vi "PPS TCP Parser's Calling or Specified VI's Clustered Controls Details.vi"(0 "Calling VI (T)":bool, 5 "Specified VI (if Calling VI = F)":path=path "Optical Prober Control v5.0.2j.vi", 11 "error in (no error)":errorcluster) -> (1 "Direct-access\ncontrols for\nrelabeling":refnum<vi>[](array[refnum]), 2 "Refs to controls on panel":refnum<vi>[](array[refnum]), 3 "Direct-access\ncontrols for\nrelabeling: captions":string[](array[string])=["Application Directory", "Direct Name 1", "Direct Position 1", "Direct Jog - 1", "Direct Jog + 1", "Direct Step (mm) 1", "Direct Halt Axis 1", "Direct Settings 1", "Direct Moving 1", "Direct New target 1", "Direct OK 1", "Direct Home Axis 1", "Direct Home Axis 2", "Direct OK 2", "Direct New target 2", "Direct Moving 2", "Direct Settings 2", "Direct Halt Axis 2", "Direct Step (mm) 2", "Direct Jog + 2", "Direct Jog - 2", "Direct Position 2", "Direct Name 2", "Direct Home Axis 3", "Direct OK 3", "Direct New target 3", "Direct Moving 3", "Direct Settings 3", "Direct Halt Axis 3", "Direct Step (mm) 3", "Direct Jog + 3", "Direct Jog - 3", "Direct Position 3", "Direct Name 3", "Direct Home Axis 4", "Direct OK 4", "Direct New target 4", "Direct Moving 4", "Direct Settings 4", "Direct Halt Axis 4", "Direct Step (mm) 4", "Direct Jog + 4", "Direct Jog - 4", "Direct Position 4", "Direct Name 4", "Direct Home Axis 5", "Direct OK 5", "Direct New target 5", "Direct Moving 5", "Direct Settings 5", "Direct Halt Axis 5", "Direct Step (mm) 5", "Direct Jog + 5", "Direct Jog - 5", "Direct Position 5", "Direct Name 5", "Direct Home Axis 6", "Direct OK 6", "Direct New target 6", "Direct Moving 6", "Direct Settings 6", "Direct Halt Axis 6", "Direct Step (mm) 6", "Direct Jog + 6", "Direct Jog - 6", "Direct Position 6", "Direct Name 6"], 4 "Names of Clusters":string[](array[string])=["error out"], 6 "Controls in\nthose clusters":string[][](array[string])=[["status", "code", "source"]], 8 "Refs to controls in clusters":refnum<vi>[][](array[refnum]), 10 "Refs to clusters":refnum<vi>[](array[refnum]), 12 "Controls directly on tab panes":string[](array[string])=["Interface", "S/N", "System no.", "Input XY bulls-eye", "Output XY bulls-eye", "Input Z bulls-eye", "RS Start", "RS Input XY:Enable", "RS Output XY:Enable", "RS Input XY:Status", "RS Output XY:Status", "RS Display Raw Data", "RS Input X:Range", "RS Input Y:Range", "RS Input Y:Step", "GS Start", "GS Display Raw Data", "I(t)", "Power Meter", "Output Z bulls-eye", "stop", "ID", "RS Frequency", "RS Input X:Center", "RS Input Y:Center", "RS Output X:Range", "RS Output Y:Range", "RS Output Y:Step", "RS Output X:Center", "RS Output Y:Center", "RS Input XY:Duration", "RS Output XY:Duration", "idle loop (msec)", "RS:Settle at 1st corner", "Axis role file", "Application Directory", "GS Status", "Power Meter Average", "RS Input XY:Swap Axes", "RS Output XY:Swap Axes", "PZT Input X:Position", "PZT Input Y:Position", "PZT Output X:Position", "PZT Output Y:Position", "PZT Input Z:Position", "PZT Output Z:Position", "RS Status", "PZT motion", "Motor motion", "Motor Input X:Name", "Motor Input X:Position", "Motor Input X:Jog +", "Motor Input X:Jog -", "Motor Input X:Step (mm)", "Motor Input X:Halt Axis", "Motor Input X:Settings", "Motor Input X:Moving", "Motor Input X:New Target", "Motor Input X:OK", "Motor Input X:Home Axis", "Motor Input Y:Home Axis", "Motor Input Y:OK", "Motor Input Y:New Target", "Motor Input Y:Moving", "Motor Input Y:Settings", "Motor Input Y:Halt Axis", "Motor Input Y:Step (mm)", "Motor Input Y:Jog -", "Motor Input Y:Jog +", "Motor Input Y:Position", "Motor Input Y:Name", "Motor Input Z:Home Axis", "Motor Input Z:OK", "Motor Input Z:New Target", "Motor Input Z:Moving", "Motor Input Z:Settings", "Motor Input Z:Halt Axis", "Motor Input Z:Step (mm)", "Motor Input Z:Jog -", "Motor Input Z:Jog +", "Motor Input Z:Position", "Motor Input Z:Name", "Motor Output X:Home Axis", "Motor Output X:OK", "Motor Output X:New Target", "Motor Output X:Moving", "Motor Output X:Settings", "Motor Output X:Halt Axis", "Motor Output X:Step (mm)", "Motor Output X:Jog -", "Motor Output X:Jog +", "Motor Output X:Position", "Motor Output X:Name", "Motor Output Y:Home Axis", "Motor Output Y:OK", "Motor Output Y:New Target", "Motor Output Y:Moving", "Motor Output Y:Settings", "Motor Output Y:Halt Axis", "Motor Output Y:Step (mm)", "Motor Output Y:Jog -", "Motor Output Y:Jog +", "Motor Output Y:Position", "Motor Output Y:Name", "Motor Output Z:Home Axis", "Motor Output Z:OK", "Motor Output Z:New Target", "Motor Output Z:Moving", "Motor Output Z:Settings", "Motor Output Z:Halt Axis", "Motor Output Z:Step (mm)", "Motor Output Z:Jog -", "Motor Output Z:Jog +", "Motor Output Z:Position", "Motor Output Z:Name", "GS Input XY:Enable", "GS Output XY:Enable", "GS Input Z:Enable", "GS Output Z:Enable", "GS Input XY:Status", "GS Output XY:Status", "GS Input Z:Status", "GS Output Z:Status", "RS Fit", "RS:Lower Clip Level", "RS:Upper Clip Level", "GS:Couple Processes", "FW", "RS Input:Successful", "GS Input XY:Success", "GS Output XY:Success", "GS Input Z:Success", "GS Output Z:Success", "RS Input:Threshold (mW)", "RS Output:Threshold (mW)", "RS Output:Successful", "Default settling window", "Scan axis center", "Step axis center", "Z axis center", "NxM Dithers", "RS Input XY:Data", "RS Output XY:Data", "error out", "Override Pane", "GS Input XY:Duration", "GS Output XY:Duration", "GS Input Z:Duration", "GS Input Z:Duration", "PZT Input X:New Target", "Scan Processes (from axis roles file)", "GS Parameters:Update", "PZT Input Y:New Target", "PZT Output X:New Target", "PZT Output Y:New Target", "PZT Output Z:New Target", "PZT Input Z:New Target", "GS Input XY:HZ", "GS Input XY:V", "GS Input XY:MDC", "GS Input XY:MINR", "GS Input XY:MAXR", "GS Input XY:ML", "GS Input XY:SP", "GS Output XY:HZ", "GS Output XY:V", "GS Output XY:MDC", "GS Output XY:MINR", "GS Output XY:MAXR", "GS Output XY:ML", "GS Output XY:SP", "GS Input Z:HZ", "GS Input Z:V", "GS Input Z:MDC", "GS Input Z:MINR", "GS Input Z:MAXR", "GS Input Z:ML", "GS Input Z:SP", "GS Output Z:HZ", "GS Output Z:V", "GS Output Z:MDC", "GS Output Z:MINR", "GS Output Z:MAXR", "GS Output Z:ML", "GS Output Z:SP", "GS Input XY process name", "GS Input XY StepAxNumber", "GS Input XY ScanAxNumber", "GS Input XY ScanAxName", "GS Input XY StepAxName", "GS Output XY process name", "GS Output XY StepAxNumber", "GS Output XY ScanAxNumber", "GS Output XY ScanAxName", "GS Output XY StepAxName", "GS Input Z process name", "GS Input Z StepAxNumber", "GS Input Z ScanAxNumber", "GS Input Z ScanAxName", "GS Input Z StepAxName", "GS Output Z process name", "GS Output Z StepAxNumber", "GS Output Z ScanAxNumber", "GS Output Z ScanAxName", "GS Output Z StepAxName", "msec timestamp"], 13 "Refs to controls directly on tab panes":refnum<vi>[](array[refnum]), 14 "Controls on panel":string[](array[string])=["Halt Homing", "Tab Control", "Names of Clusters", "Controls in clusters", "Refs to clusters", "PZT Input X:OK", "PZT Input Y:OK", "PZT Input Z:OK", "PZT Output X:OK", "PZT Output Y:OK", "PZT Output Z:OK"], 15 "error out":errorcluster)   [LabVIEW 2016]
panel:
  out "Array":string[](array[string])=["Array", "Array", "Array"]
  out "Arrays":string[](array[string])=["Names of Clusters", "Controls in clusters", "Refs to clusters"]
  out "Refs to arrays":refnum<vi>[](array[refnum])
  out "Names of TabControls":string[](array[string])=["Tab Control"]
  out "Refs to TabControls":refnum<vi>[](array[refnum])
  out "Types of Controls\non panel":string[](array[string])=["Boolean", "TabControl", "Array", "Array", "Array", "Boolean", "Boolean", "Boolean", "Boolean", "Boolean", "Boolean"]
  # "This subVI finds the controls that exist on the front panel of the calling VI (OR a \nspecified VI), then selects just-the-clusters from that list.  It then finds the elements of each cluster.\n\nIF the calling VI has tab controls, the structure of this VI must accommodate the number of pages for each tab control.  Here we have nine configurations: 2-10 pages.  Add to these as necessary to accommodate the configuration of the calling VI.\n\nThis VI does not handle calling VIs with tab controls containing tab controls containing clusters...\n\nSee further discussion in the block diagram."
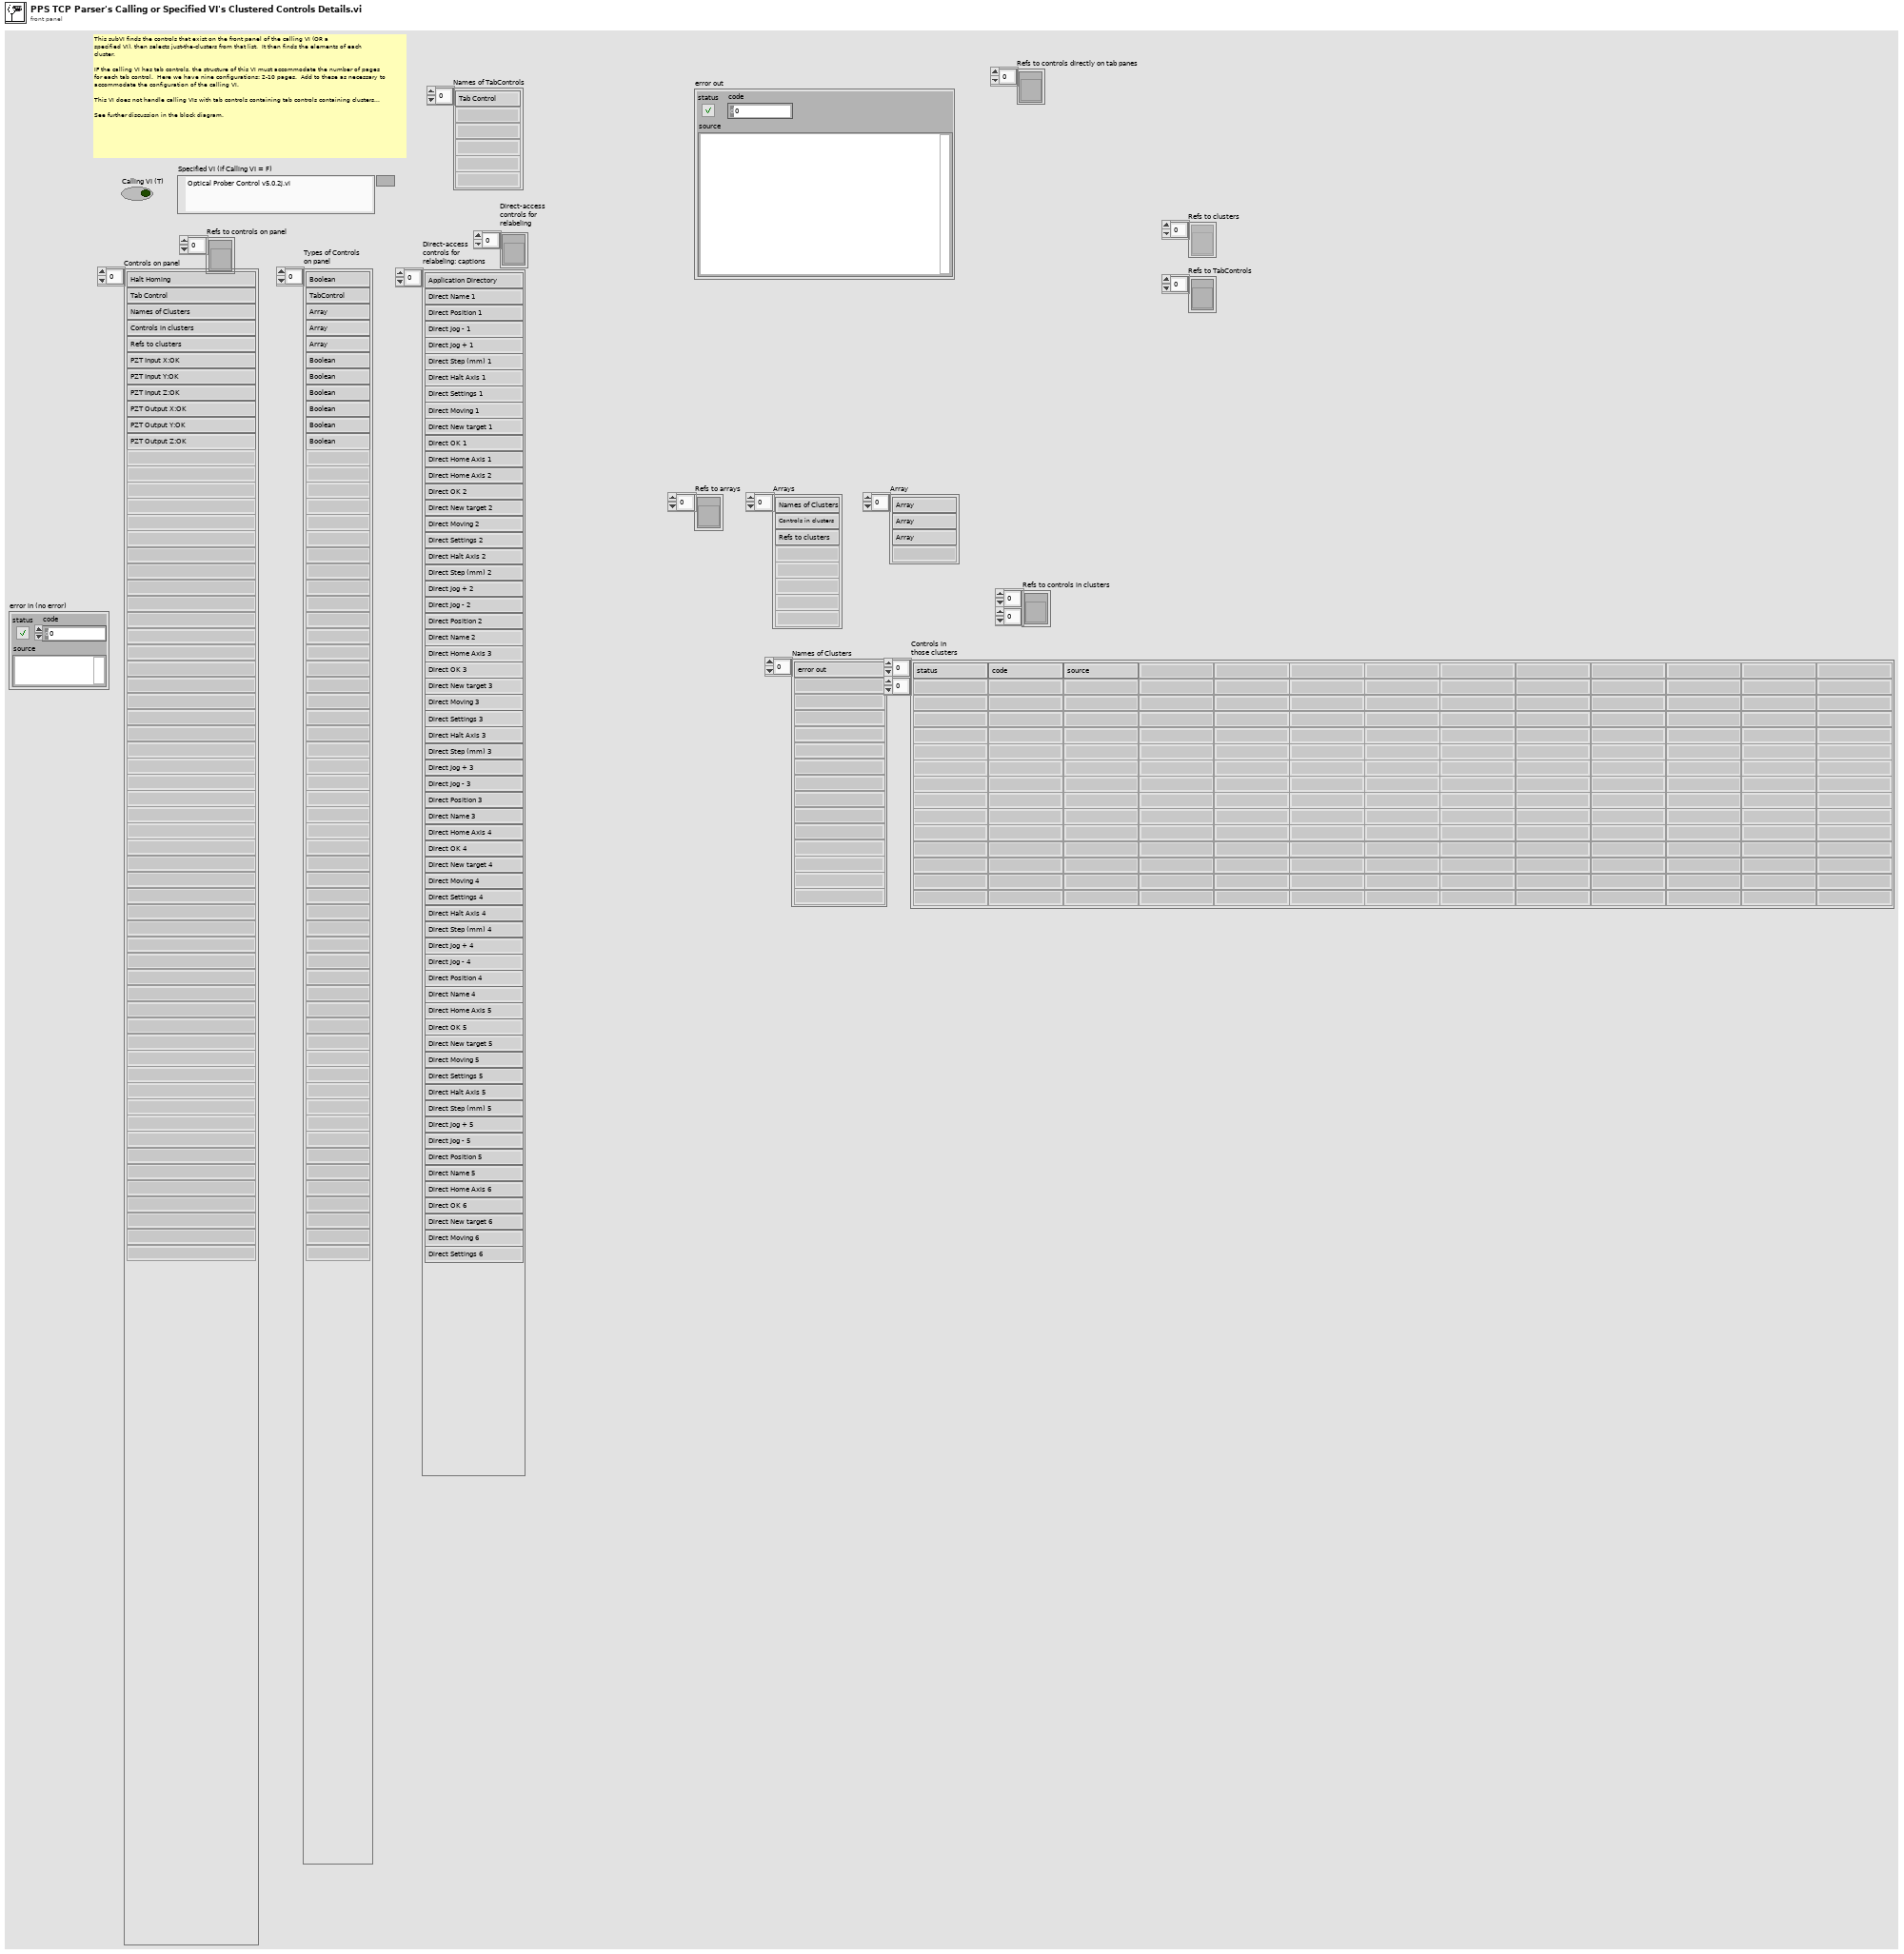
[diagram p1: front panel]
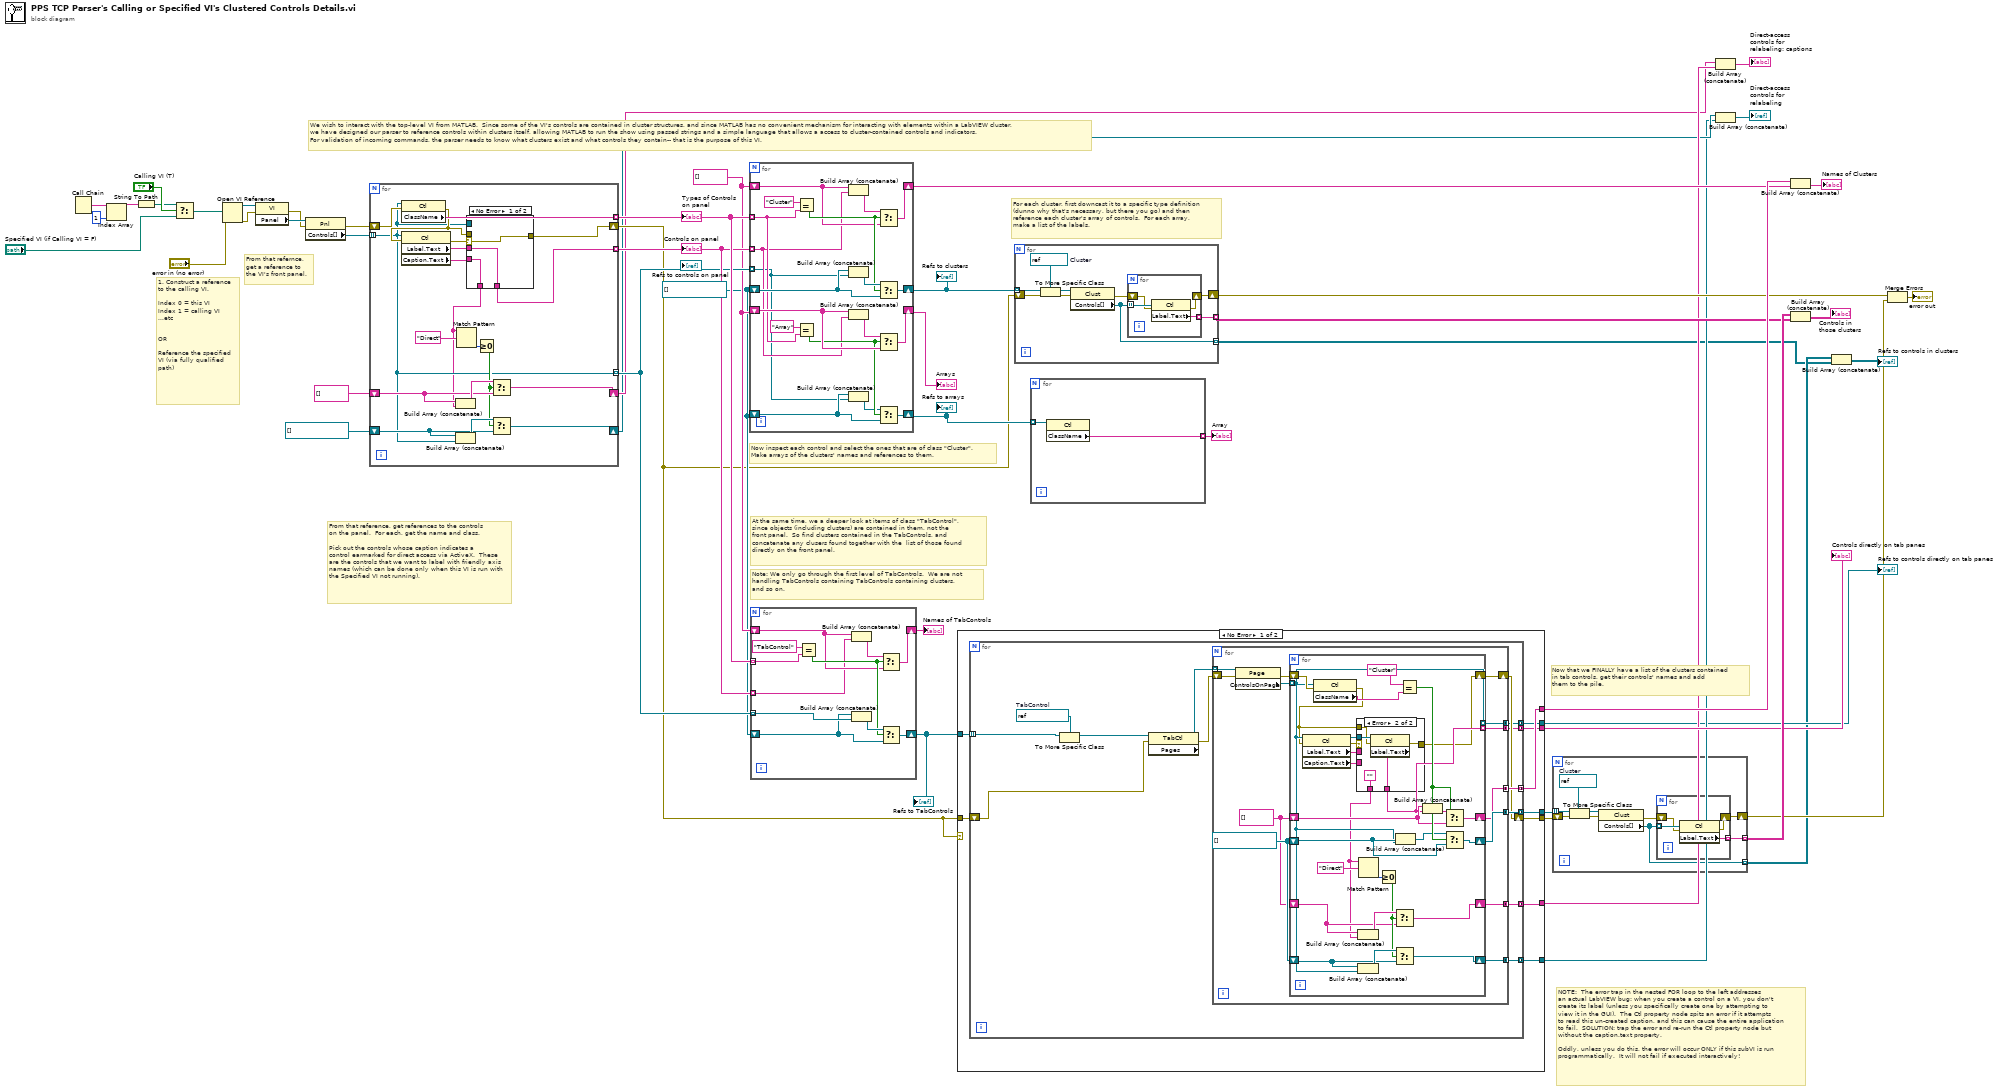
[diagram p0: block diagram]
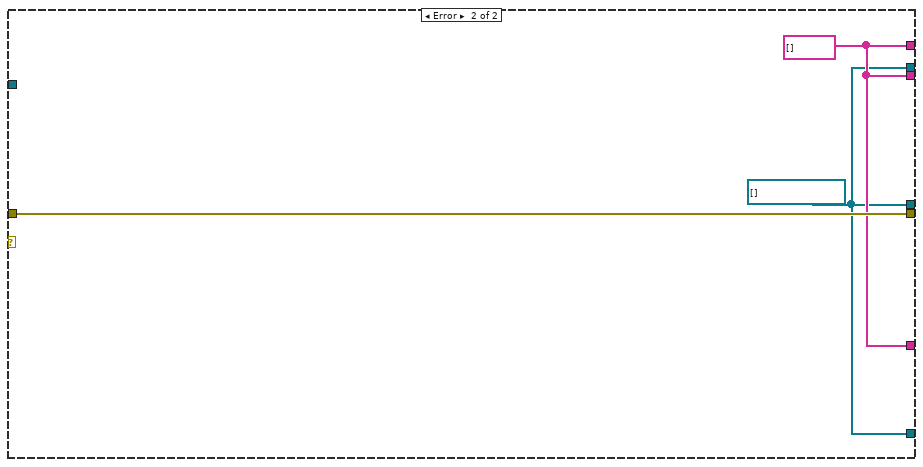
[diagram p3: hidden frame]
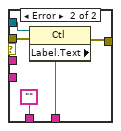
[diagram p4: hidden frame]
diagram:
  w23 = refnum<vi>[] []
  w24 = string[] []
  # "NOTE:  The error trap in the nested FOR loop to the left addresses\nan actual LabVIEW bug: when you create a control on a VI, you don't\ncreate its label (unless you specifically create one by attempting to \nview it in the GUI).  The Ctl property node spits an error if it attempts \nto read this un-created caption, and this can cause the entire application\nto fail.  SOLUTION: trap the error and re-run the Ctl property node but\nwithout the caption.text property.\n\nOddly, unless you do this, the error will occur ONLY if this subVI is run\nprogrammatically.  It will not fail if executed interactively!"
  # "We wish to interact with the top-level VI from MATLAB.  Since some of the VI's controls are contained in cluster structures, and since MATLAB has no convenient mechanism for interacting with elements within a LabVIEW cluster, \nwe have designed our parser to reference controls within clusters itself, allowing MATLAB to run the show using passed strings and a simple language that allows a access to cluster-contained controls and indicators.  \nFor validation of incoming commands, the parser needs to know what clusters exist and what controls they contain-- that is the purpose of this VI."
  # "Now that we FINALLY have a list of the clusters contained\nin tab controls, get their controls' names and add \nthem to the pile."
  # "Note: We only go through the first level of TabControls.  We are not\nhandling TabControls containing TabControls containing clusters,\nand so on."
  # "At the same time, we a deeper look at items of class \"TabControl\", \nsince objects (including clusters) are contained in them, not the\nfront panel.  So find clusters contained in the TabControls, and \nconcatenate any clusers found together with the  list of those found \ndirectly on the front panel."
  # "For each cluster, first downcast it to a specific type definition\n(dunno why that's necessary, but there you go) and then\nreference each cluster's array of controls.  For each array,\nmake a list of the labels."
  # "Now inspect each control and select the ones that are of class \"Cluster\".\nMake arrays of the clusters' names and references to them."
  # "From that reference, get references to the controls\non the panel.  For each, get the name and class.\n\nPick out the controls whose caption indicates a \ncontrol earmarked for direct access via ActiveX.  These are the controls that we want to label with friendly axis names (which can be done only when this VI is run with the Specified VI not running)."
  # "From that refernce,\nget a reference to\nthe VI's front panel."
  # "1. Construct a reference\nto the calling VI.  \n\nIndex 0 = this VI\nIndex 1 = calling VI\n...etc\n\n\nOR\n\nReference the specified\nVI (via fully qualified\npath)"
  n1 = Call Chain() -> (call chain=w47:string[])
  n2 = Index Array(array=w47, index=1) -> (element=w18:string)
  n3 = String To Path(string=w18) -> (path=w15:path)
  n4 = Select(t=w15, s="Calling VI (T)", f="Specified VI (if Calling VI = F)") -> (s? t:f=w17:path)
  n5 = Open VI Reference(vi path=w17, error in (no error)="error in (no error)") -> (vi reference=w45:refnum<vi>, error out=w43:errorcluster)  [unwired: 4 in]
  n6 = property class="VI"(reference=w45, error in=w43) -> (error out=w42:errorcluster, "Panel"=w50:refnum<vi>)  [unwired: 1 out]
  n7 = property class="Pnl"(reference=w50, error in=w42) -> (error out=w41:errorcluster, "Controls[]"=w49:refnum<vi>[])  [unwired: 1 out]
  n8 = for {
    tunnel: w49 -> [w55] mode=indexing
    tunnel: [w52] -> w38 mode=indexing
    tunnel: [w69] -> w39 mode=indexing
    tunnel: [w55] -> w37 mode=indexing
    shift-right: [w57] -> w11
    shift-left: w41 -> [w68]
    shift-right: [w67] -> w9
    shift-left: string[] [] -> [w65]
    shift-right: [w63] -> w7
    shift-left: refnum<vi>[] [] -> [w62]
    n9 = property class="Ctl"(reference=w55, error in=w68) -> (error out=w56:errorcluster, "ClassName"=w69:string)  [unwired: 1 out]
    n10 = property class="Ctl"(reference=w55, error in=w56) -> (error out=w58:errorcluster, "Label.Text"=w54:string, "Caption.Text"=w53:string)  [unwired: 1 out]
    n11 = Build Array (concatenate)(w62, w55) -> (w64:refnum<vi>[])
    n12 = case shown="No Error" w58 {
      selector: w58 -> [w71 _]
      tunnel: w56 -> [_ w73]
      tunnel: w54 -> [w72 _]
      tunnel: [w72 w77] -> w52
      tunnel: w55 -> [_ w74]
      tunnel: [w71 w75] -> w57
      tunnel: [w70 ""] -> w51
      tunnel: w53 -> [w70 _]
      frame No Error {
      }
      frame Error {
        n13 = property class="Ctl"(reference=w74, error in=w73) -> (error out=w75:errorcluster, "Label.Text"=w77:string)  [unwired: 1 out]
      }
    }
    n14 = Build Array (concatenate)(w65, w51) -> (w66:string[])
    n15 = Match Pattern(string=w51, regular expression="Direct") -> (offset past match=w60:i32)  [unwired: 1 in, 3 out]
    n16 = Greater Or Equal To 0?(x=w60) -> (x >= 0?=w59:bool)
    n17 = Select(t=w66, s=w59, f=w65) -> (s? t:f=w67:string[])
    n18 = Select(t=w64, s=w59, f=w62) -> (s? t:f=w63:refnum<vi>[])
  }
  "Controls on panel" <- w38
  "Types of Controls\non panel" <- w39
  "Refs to controls on panel" <- w37
  n19 = for {
    tunnel: w39 -> [w81] mode=indexing
    tunnel: w38 -> [w80] mode=indexing
    shift-right: [w94] -> w31
    shift-left: w24 -> [w90]
    tunnel: w37 -> [w79] mode=indexing
    shift-right: [w92] -> w48
    shift-left: w23 -> [w89]
    shift-right: [w78] -> w22
    shift-left: w24 -> [w87]
    shift-right: [w85] -> w21
    shift-left: w23 -> [w88]
    n20 = Equal?(x="Cluster", y=w81) -> (x = y?=w91:bool)
    n21 = Equal?(x="Array", y=w81) -> (x = y?=w86:bool)
    n22 = Build Array (concatenate)(w90, w80) -> (w95:string[])
    n23 = Build Array (concatenate)(w89, w79) -> (w93:refnum<vi>[])
    n24 = Build Array (concatenate)(w87, w80) -> (w83:string[])
    n25 = Build Array (concatenate)(w88, w79) -> (w84:refnum<vi>[])
    n26 = Select(t=w95, s=w91, f=w90) -> (s? t:f=w94:string[])
    n27 = Select(t=w93, s=w91, f=w89) -> (s? t:f=w92:refnum<vi>[])
    n28 = Select(t=w83, s=w86, f=w87) -> (s? t:f=w78:string[])
    n29 = Select(t=w84, s=w86, f=w88) -> (s? t:f=w85:refnum<vi>[])
  }
  "Refs to clusters" <- w48
  "Refs to arrays" <- w21
  "Arrays" <- w22
  n30 = for {
    tunnel: w39 -> [w107] mode=indexing
    tunnel: w38 -> [w99] mode=indexing
    shift-right: [w104] -> w40
    shift-left: w24 -> [w100]
    tunnel: w37 -> [w98] mode=indexing
    shift-right: [w102] -> w36
    shift-left: w23 -> [w97]
    n31 = Equal?(x="TabControl", y=w107) -> (x = y?=w101:bool)
    n32 = Build Array (concatenate)(w100, w99) -> (w105:string[])
    n33 = Build Array (concatenate)(w97, w98) -> (w103:refnum<vi>[])
    n34 = Select(t=w105, s=w101, f=w100) -> (s? t:f=w104:string[])
    n35 = Select(t=w103, s=w101, f=w97) -> (s? t:f=w102:refnum<vi>[])
  }
  "Names of TabControls" <- w40
  "Refs to TabControls" <- w36
  n36 = case shown="No Error" w11 {
    tunnel: w36 -> [w116 _]
    tunnel: [w115 w179] -> w35
    tunnel: [w114 w180] -> w32
    tunnel: [w113 w181] -> w28
    tunnel: w11 -> [w112 w181]
    tunnel: [w111 w180] -> w19
    tunnel: [w110 w180] -> w10
    tunnel: [w109 w179] -> w6
    tunnel: [w108 w179] -> w4
    frame No Error {
      n37 = for {
        tunnel: w116 -> [w119] mode=indexing
        tunnel: [w128] -> w115 mode=concatenating
        tunnel: [w127] -> w114 mode=concatenating
        shift-right: [w125] -> w113
        shift-left: w112 -> [w120]
        tunnel: [w124] -> w111 mode=concatenating
        tunnel: [w123] -> w110 mode=concatenating
        tunnel: [w122] -> w109 mode=concatenating
        tunnel: [w121] -> w108 mode=concatenating
        w117 = refnum<vi> refnum  # TabControl
        n38 = To More Specific Class(target class=w117, reference=w119) -> (specific class reference=w118:refnum<vi>)  [unwired: 1 in, 1 out]
        n39 = property class="TabCtl"(reference=w118, error in=w120) -> (error out=w126:errorcluster, "Pages"=w129:refnum<vi>[])  [unwired: 1 out]
        n40 = for {
          tunnel: w129 -> [w142] mode=indexing
          tunnel: [w140] -> w128 mode=concatenating
          tunnel: [w139] -> w127 mode=concatenating
          shift-right: [w136] -> w125
          shift-left: w126 -> [w138]
          tunnel: [w135] -> w124 mode=concatenating
          tunnel: [w132] -> w123 mode=concatenating
          tunnel: [w131] -> w122 mode=concatenating
          tunnel: [w130] -> w121 mode=concatenating
          w133 = string[] []
          w134 = refnum<vi>[] []
          n41 = property class="Page"(reference=w142, error in=w138) -> (error out=w137:errorcluster, "ControlsOnPage"=w141:refnum<vi>[])  [unwired: 1 out]
          n42 = for {
            tunnel: w141 -> [w151] mode=indexing
            shift-right: [w167] -> w139
            shift-left: w133 -> [w163]
            shift-right: [w164] -> w140
            shift-left: w134 -> [w162]
            shift-right: [w145] -> w136
            shift-left: w137 -> [w161]
            tunnel: [w147] -> w135 mode=indexing
            shift-right: [w152] -> w131
            shift-left: w134 -> [w153]
            shift-right: [w154] -> w132
            shift-left: w133 -> [w155]
            tunnel: [w151] -> w130 mode=indexing
            n43 = property class="Ctl"(reference=w151, error in=w161) -> (error out=w146:errorcluster, "ClassName"=w169:string)  [unwired: 1 out]
            n44 = property class="Ctl"(reference=w151, error in=w146) -> (reference out=w149:refnum<vi>, error out=w150:errorcluster, "Label.Text"=w148:string, "Caption.Text"=w143:string)
            n45 = case shown="Error" w150 {
              selector: w150 -> [w172 _]
              tunnel: w149 -> [_ w178]
              tunnel: w148 -> [w173 _]
              tunnel: [w173 w176] -> w147
              tunnel: w146 -> [_ w177]
              tunnel: [w172 w174] -> w145
              tunnel: [w171 ""] -> w144
              tunnel: w143 -> [w171 _]
              frame No Error {
              }
              frame Error {
                n46 = property class="Ctl"(reference=w178, error in=w177) -> (error out=w174:errorcluster, "Label.Text"=w176:string)  [unwired: 1 out]
              }
            }
            n47 = Build Array (concatenate)(w155, w144) -> (w160:string[])
            n48 = Build Array (concatenate)(w153, w151) -> (w159:refnum<vi>[])
            n49 = Match Pattern(string=w144, regular expression="Direct") -> (offset past match=w157:i32)  [unwired: 1 in, 3 out]
            n50 = Greater Or Equal To 0?(x=w157) -> (x >= 0?=w156:bool)
            n51 = Select(t=w160, s=w156, f=w155) -> (s? t:f=w154:string[])
            n52 = Select(t=w159, s=w156, f=w153) -> (s? t:f=w152:refnum<vi>[])
            n53 = Build Array (concatenate)(w162, w151) -> (w165:refnum<vi>[])
            n54 = Equal?(x="Cluster", y=w169) -> (x = y?=w166:bool)
            n55 = Build Array (concatenate)(w163, w147) -> (w168:string[])
            n56 = Select(t=w168, s=w166, f=w163) -> (s? t:f=w167:string[])
            n57 = Select(t=w165, s=w166, f=w162) -> (s? t:f=w164:refnum<vi>[])
          }
        }
      }
    }
    frame Error {
      w180 = string[] []
      w179 = refnum<vi>[] []
    }
  }
  "Controls directly on tab panes" <- w19
  "Refs to controls directly on tab panes" <- w4
  n58 = for {
    tunnel: w48 -> [w190] mode=indexing
    tunnel: [w187] -> w29 mode=indexing
    shift-right: [w183] -> w26
    shift-left: w11 -> [w186]
    tunnel: [w182] -> w1 mode=indexing
    w189 = refnum<vi> refnum  # Cluster
    n59 = To More Specific Class(target class=w189, reference=w190, error in=w186) -> (specific class reference=w188:refnum<vi>, error out=w185:errorcluster)
    n60 = property class="Clust"(reference=w188, error in=w185) -> (error out=w184:errorcluster, "Controls[]"=w182:refnum<vi>[])  [unwired: 1 out]
    n61 = for {
      tunnel: w182 -> [w194] mode=indexing
      tunnel: [w193] -> w187 mode=indexing
      shift-right: [w191] -> w183
      shift-left: w184 -> [w192]
      n62 = property class="Ctl"(reference=w194, error in=w192) -> (error out=w191:errorcluster, "Label.Text"=w193:string)  [unwired: 1 out]
    }
  }
  n63 = for {
    tunnel: w21 -> [w196] mode=indexing
    tunnel: [w195] -> w20 mode=indexing
    n64 = property class="Ctl"(reference=w196) -> ("ClassName"=w195:string)  [unwired: 1 in, 2 out]
  }
  "Array" <- w20
  n65 = for {
    tunnel: w35 -> [w205] mode=indexing
    tunnel: [w202] -> w30 mode=indexing
    shift-right: [w198] -> w25
    shift-left: w28 -> [w201]
    tunnel: [w197] -> w2 mode=indexing
    w204 = refnum<vi> refnum  # Cluster
    n66 = To More Specific Class(target class=w204, reference=w205, error in=w201) -> (specific class reference=w203:refnum<vi>, error out=w200:errorcluster)
    n67 = property class="Clust"(reference=w203, error in=w200) -> (error out=w199:errorcluster, "Controls[]"=w197:refnum<vi>[])  [unwired: 1 out]
    n68 = for {
      tunnel: w197 -> [w209] mode=indexing
      tunnel: [w208] -> w202 mode=indexing
      shift-right: [w206] -> w198
      shift-left: w199 -> [w207]
      n69 = property class="Ctl"(reference=w209, error in=w207) -> (error out=w206:errorcluster, "Label.Text"=w208:string)  [unwired: 1 out]
    }
  }
  n70 = Build Array (concatenate)(w9, w10) -> (→"Direct-access\ncontrols for\nrelabeling: captions":string[])
  n71 = Build Array (concatenate)(w7, w6) -> (→"Direct-access\ncontrols for\nrelabeling":refnum<vi>[])
  n72 = Build Array (concatenate)(w32, w31) -> (→"Names of Clusters":string[])
  n73 = Build Array (concatenate)(w30, w29) -> (→"Controls in\nthose clusters":string[][])
  n74 = Build Array (concatenate)(w2, w1) -> (→"Refs to controls in clusters":refnum<vi>[][])
  n75 = Merge Errors(w26, w25) -> (→"error out":errorcluster)
